vi "spectrum_example.vi"() -> ()   [LabVIEW 2017]
uses:
  <userlib>/RSA_API/RSA_API.lvlib
  <vilib>/Analysis/NI_AALBase.lvlib
  <vilib>/Analysis/1siggen.llb/Ramp Pattern by Samples.vi
panel:
  in  "settings":T1={"span"=80000000.0, "rbw"=500.0, "enableVBW"=FALSE, "vbw"=0.0, "traceLength"=0, "window"=0, "verticalUnit"=0, "actualStartFreq"=0.0, "actualStopFreq"=0.0, "actualFreqStepSize"=0.0, "actualRBW"=0.0, "actualVBW"=0.0, "actualNumIQSamples"=0} {"window" items=["SpectrumWindow_Kaiser", "SpectrumWindow_Mil6dB", "SpectrumWindow_BlackmanHarris", "SpectrumWindow_Rectangle", "SpectrumWindow_FlatTop", "SpectrumWindow_Hann"]; "verticalUnit" items=["SpectrumVerticalUnit_dBm", "SpectrumVerticalUnit_Watt", "SpectrumVerticalUnit_Volt", "SpectrumVerticalUnit_Amp", "SpectrumVerticalUnit_dBmV"]}
  out "rbwOut":dbl format="%#_13g"
  out "spanOut":dbl format="%#_13g"
  out "refLevelOut":dbl
  out "cfOut":dbl
  out "SpectrumEnableOut":bool
  out "XY Graph":T2(graph)
  out "TraceReady":bool
  in  "refLevelIn":dbl
  in  "cfIn":dbl
  in  "deviceID":i32
  out "deviceType":string
  out "deviceSerial":string
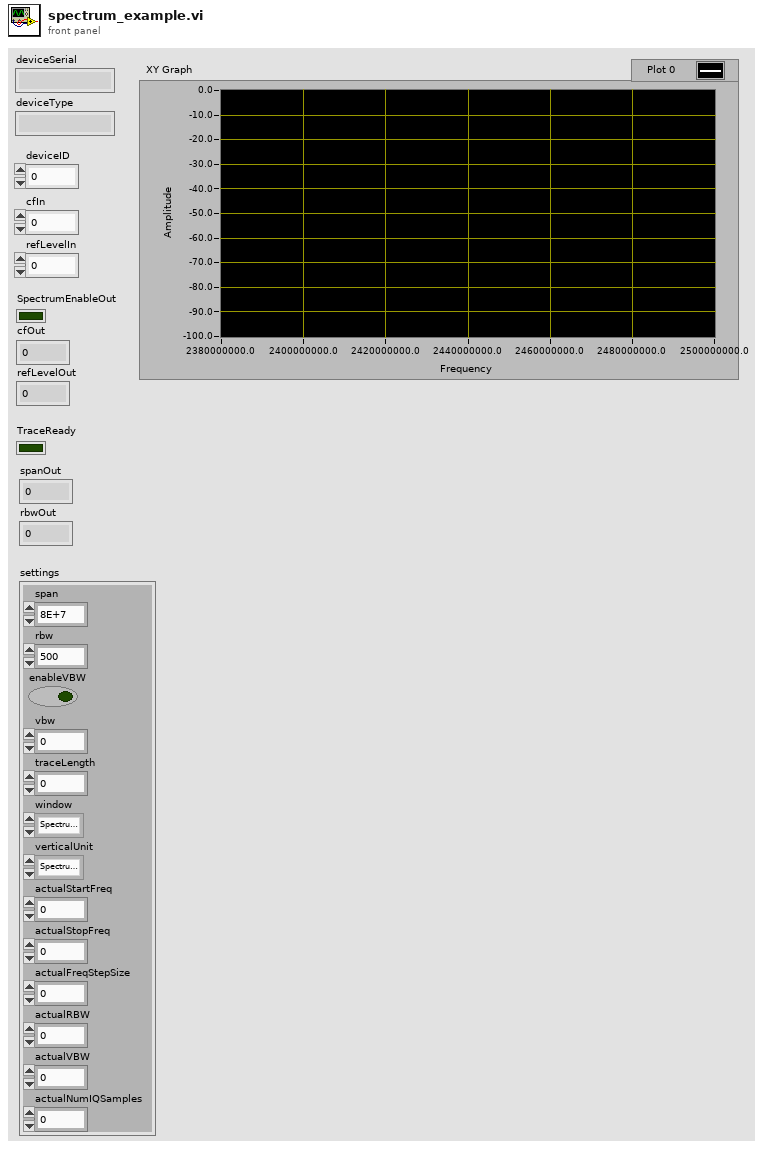
[diagram p1: front panel]
types:
  T1 = cluster{"span":dbl, "rbw":dbl, "enableVBW":bool, "vbw":dbl, "traceLength":i32, "window":u32, "verticalUnit":u32, "actualStartFreq":dbl, "actualStopFreq":dbl, "actualFreqStepSize":dbl, "actualRBW":dbl, "actualVBW":dbl, "actualNumIQSamples":i32}
  T2 = cluster{"Ramp Pattern":dbl[], "traceData out":sgl[]}
  T3 = cluster{"Ramp Pattern":dbl[], "traceData out":sgl}
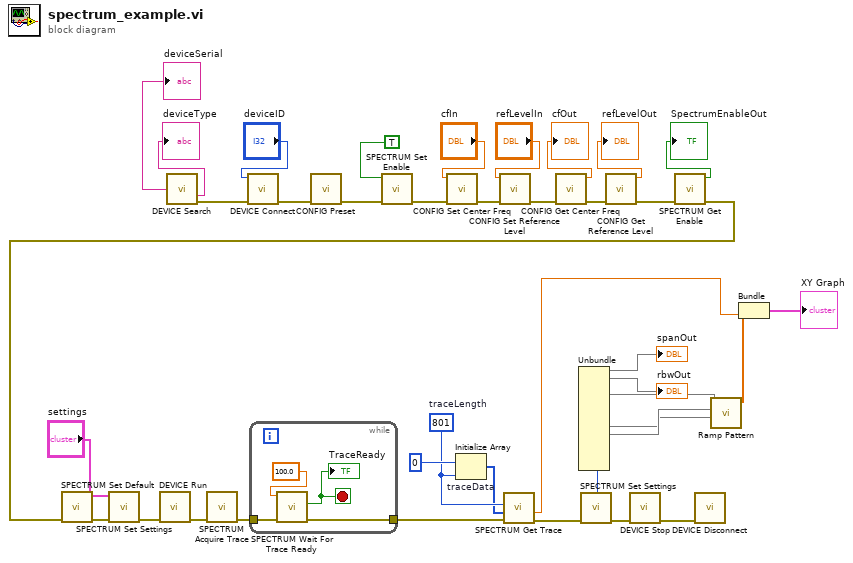
[diagram p0: block diagram]
diagram:
  w27 = 801  # traceLength
  n1 = call <userlib>:"DEVICE Search.vi"() -> ("deviceSerial out"=→"deviceSerial":string, "deviceType out"=→"deviceType":string, "error out"=w37:errorcluster)  [unwired: 10 in, 3 out]
  n2 = call <userlib>:"DEVICE Connect.vi"("error in (no error)"=w37, "deviceID"="deviceID") -> ("error out"=w35:errorcluster)  [unwired: 8 in, 1 out]
  n3 = call <userlib>:"CONFIG Preset.vi"("error in (no error)"=w35) -> ("error out"=w32:errorcluster)  [unwired: 9 in, 1 out]
  n4 = call <userlib>:"SPECTRUM Set Enable.vi"("error in (no error)"=w32, "enable"=TRUE) -> ("error out"=w25:errorcluster)  [unwired: 8 in, 1 out]
  n5 = call <userlib>:"CONFIG Set Center Freq.vi"("error in (no error)"=w25, "cf"="cfIn") -> ("error out"=w24:errorcluster)  [unwired: 8 in, 1 out]
  n6 = Initialize Array "traceData"(0, w27) -> (w13:i32[])
  n7 = call <userlib>:"CONFIG Set Reference Level.vi"("error in (no error)"=w24, "refLevel"="refLevelIn") -> ("error out"=w20:errorcluster)  [unwired: 8 in, 1 out]
  n8 = call <userlib>:"CONFIG Get Center Freq.vi"("error in (no error)"=w20) -> ("error out"=w19:errorcluster, "cf out"=→"cfOut":dbl)  [unwired: 8 in, 1 out]
  n9 = call <userlib>:"CONFIG Get Reference Level.vi"("error in (no error)"=w19) -> ("error out"=w18:errorcluster, "refLevel out"=→"refLevelOut":dbl)  [unwired: 8 in, 1 out]
  n10 = call <userlib>:"SPECTRUM Get Enable.vi"("error in (no error)"=w18) -> ("error out"=w17:errorcluster, "enable out"=→"SpectrumEnableOut":bool)  [unwired: 8 in, 1 out]
  n11 = call <userlib>:"SPECTRUM Set Default.vi"("error in (no error)"=w17) -> ("error out"=w8:errorcluster)  [unwired: 9 in, 1 out]
  n12 = call <userlib>:"SPECTRUM Set Settings.vi"("error in (no error)"=w8, "settings"="settings") -> ("error out"=w7:errorcluster)  [unwired: 8 in, 1 out]
  n13 = call <userlib>:"DEVICE Run.vi"("error in (no error)"=w7) -> ("error out"=w30:errorcluster)  [unwired: 9 in, 1 out]
  n14 = call <userlib>:"SPECTRUM Acquire Trace.vi"("error in (no error)"=w30) -> ("error out"=w29:errorcluster)  [unwired: 9 in, 1 out]
  n15 = while {
    tunnel: [w43] -> w12
    tunnel: w29 -> [w42]
    stop <- w40 stop-if-true
    n16 = call <userlib>:"SPECTRUM Wait For Trace Ready.vi"("error in (no error)"=w42, "timeoutMsec"=100.0) -> ("error out"=w43:errorcluster, "ready out"=w40:bool)  [unwired: 7 in, 1 out]
    "TraceReady" <- w40
  }
  n17 = call <userlib>:"SPECTRUM Get Trace.vi"("error in (no error)"=w12, "traceData"=w13, "maxTracePoints"=w27) -> ("error out"=w11:errorcluster, "traceData out"=w10:sgl)  [unwired: 5 in, 2 out]
  n18 = call <userlib>:"SPECTRUM Set Settings.vi"("error in (no error)"=w11) -> ("error out"=w9:errorcluster, "function return"=w31:u32)  [unwired: 9 in]
  n19 = Unbundle(w31) -> (→"spanOut", →"rbwOut", w1, w2, w3)  [unwired: 8 out]
  n20 = call <userlib>:"DEVICE Stop.vi"("error in (no error)"=w9) -> ("error out"=w26:errorcluster)  [unwired: 9 in, 1 out]
  n21 = call <userlib>:"DEVICE Disconnect.vi"("error in (no error)"=w26) -> ()  [unwired: 9 in, 2 out]
  n22 = call-poly <vilib>:"Ramp Pattern.vi"("start"=w2, "end"=w3, "samples"=w1) -> ("Ramp Pattern"=w22:dbl[])  [unwired: 7 in, 1 out]
  n23 = Bundle("Ramp Pattern"=w22, "traceData out"=w10) -> (→"XY Graph":T3)  [unwired: 1 in]
